vi "Open Motors.vi"(9 "PID Constants":T6={"P Gain"=0.0, "I Gain"=0.0, "D Gain"=0.0, "F Gain"=0.0, "I Zone"=0.0, "Min Output"=-1.0, "Max Output"=1.0}) -> (0 "error out":errorcluster, 1 "Right":T1={"DeviceStatus"={"status"=FALSE, "code"=0, "source"=""}, "Type"=enum."PWM", "PWM"={"PWM Channel"=enum."Invalid", "DeadBand"={"Name"="", "maxPositivePwm"=0, "minPositivePwm"=0, "centerPwm"=0, "maxNegativePwm"=0, "minNegativePwm"=0, "angularRange"=0}}, "CAN"={"Device Number"=0, "SetOutput VI Ref"=variant(refnum<vi> refnum), "GetOutput VI Ref"=variant(refnum<vi> refnum), "Enable VI Ref"=variant(refnum<vi> refnum), "Disable VI Ref"=variant(refnum<vi> refnum), "Data"=variant}, "Invert"=FALSE, "DIO PWM"={"PWM \"Enable\" Channel"=enum."Invalid", "DIOChannel"=enum."Invalid", "PWM Rate"=0.0}}, 2 "Left":T1={"DeviceStatus"={"status"=FALSE, "code"=0, "source"=""}, "Type"=enum."PWM", "PWM"={"PWM Channel"=enum."Invalid", "DeadBand"={"Name"="", "maxPositivePwm"=0, "minPositivePwm"=0, "centerPwm"=0, "maxNegativePwm"=0, "minNegativePwm"=0, "angularRange"=0}}, "CAN"={"Device Number"=0, "SetOutput VI Ref"=variant(refnum<vi> refnum), "GetOutput VI Ref"=variant(refnum<vi> refnum), "Enable VI Ref"=variant(refnum<vi> refnum), "Disable VI Ref"=variant(refnum<vi> refnum), "Data"=variant}, "Invert"=FALSE, "DIO PWM"={"PWM \"Enable\" Channel"=enum."Invalid", "DIOChannel"=enum."Invalid", "PWM Rate"=0.0}}, 3 "WPI Robot":T7={"DevStatus"={"status"=FALSE, "code"=0, "source"=""}, "Motors[]"=[], "Square Inputs"=FALSE, "Max Output"=1.0})   [LabVIEW 2018]
uses:
  <vilib>/Rock Robotics/WPI/RobotDrive/WPI_RobotDriveDevRef.ctl
  <vilib>/Rock Robotics/WPI/MotorControl/WPI_MotorControlDeviceRef.ctl
  <vilib>/Rock Robotics/WPI/MotorControl/WPI_MotorControlType.ctl
  <vilib>/Rock Robotics/SystemInterfaces/DIO/FPGA_DIOPWMChannel.ctl
  <vilib>/Rock Robotics/WPI/PWM/WPI_PWMDeadband.ctl
  <vilib>/Rock Robotics/SystemInterfaces/DIO/FPGA_DIOChannel.ctl
  <vilib>/Rock Robotics/WPI/SafetyOutput/WPI_SafetyOutputConfigMenu.ctl
  <vilib>/Rock Robotics/WPI/ThirdParty/REV Robotics/SPARK MAX/Typedef/Spark MAX Motor Type.ctl
  <vilib>/Rock Robotics/WPI/RobotDrive/WPI_RobotDriveOpen2MotorWithExistingMotors.vi
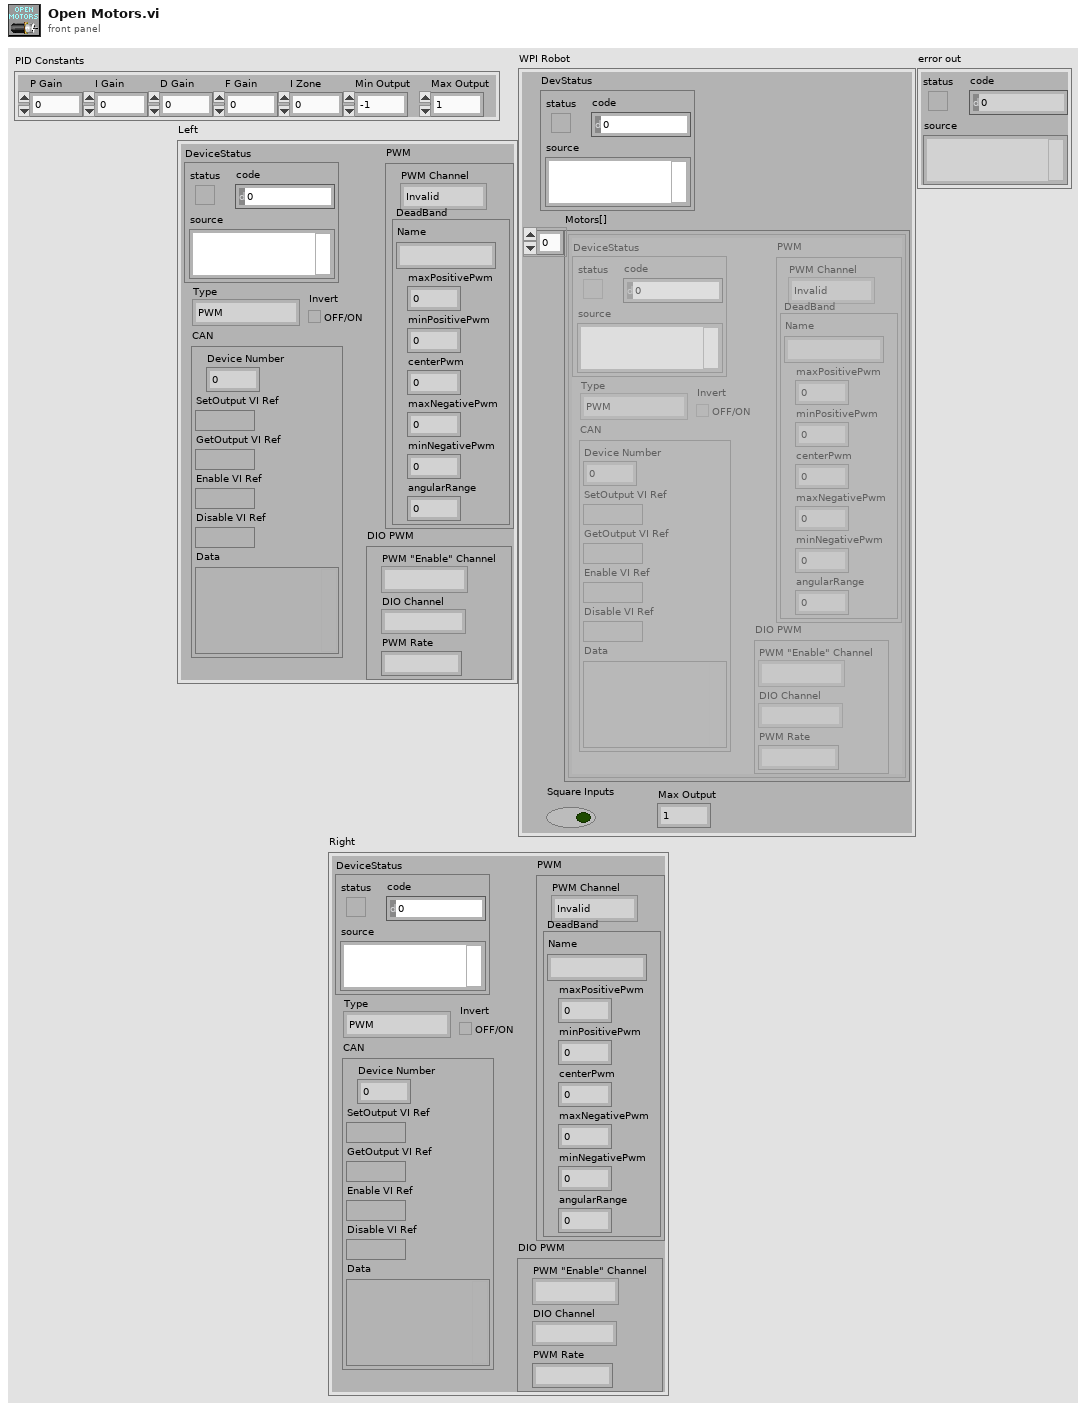
[diagram p1: front panel]
types:
  T1 = typedef "WPI_MotorControlDeviceRef.ctl" = cluster{"DeviceStatus":errorcluster, "Type":T2, "PWM":cluster{"PWM Channel":T3, "DeadBand":T4}, "CAN":cluster{"Device Number":u8, "SetOutput VI Ref":variant, "GetOutput VI Ref":variant, "Enable VI Ref":variant, "Disable VI Ref":variant, "Data":variant}, "Invert":bool, "DIO PWM":cluster{"PWM \"Enable\" Channel":T3, "DIOChannel":T5, "PWM Rate":dbl}}
  T2 = typedef "WPI_MotorControlType.ctl" = enum16{"PWM", "CAN", "DIO PWM"}
  T3 = typedef "FPGA_DIOPWMChannel.ctl" = enum8{"PWM 0", "PWM 1", "PWM 2", "PWM 3", "PWM 4", "PWM 5", "PWM 6", "PWM 7", "PWM 8", "PWM 9", "PWM MXP 0", "PWM MXP 1", "PWM MXP 2", "PWM MXP 3", "PWM MXP 4", "PWM MXP 5", "PWM MXP 6", "PWM MXP 7", "PWM MXP 8", "PWM MXP 9", "Invalid"}
  T4 = typedef "WPI_PWMDeadband.ctl" = cluster{"Name":string, "maxPositivePwm":i32, "minPositivePwm":i32, "centerPwm":i32, "maxNegativePwm":i32, "minNegativePwm":i32, "angularRange":u16}
  T5 = typedef "FPGA_DIOChannel.ctl" = enum8{"DIO 0", "DIO 1", "DIO 2", "DIO 3", "DIO 4", "DIO 5", "DIO 6", "DIO 7", "DIO 8", "DIO 9", "DIO MXP 0", "DIO MXP 1", "DIO MXP 2", "DIO MXP 3", "DIO MXP 4", "DIO MXP 5", "DIO MXP 6", "DIO MXP 7", "DIO MXP 8", "DIO MXP 9", "DIO MXP 10", "DIO MXP 11", "DIO MXP 12", "DIO MXP 13", "DIO MXP 14", "DIO MXP 15", "SPI Port CS1", "SPI Port CS2", "SPI Port CS3", "SPI Port MISO", "SPI Port MOSI", "Invalid"}
  T6 = cluster{"P Gain":dbl, "I Gain":dbl, "D Gain":dbl, "F Gain":dbl, "I Zone":dbl, "Min Output":dbl, "Max Output":dbl}
  T7 = typedef "WPI_RobotDriveDevRef.ctl" = cluster{"DevStatus":errorcluster, "Motors[]":T1[], "Square Inputs":bool, "Max Output":dbl}
  T8 = typedef "Spark MAX Motor Type.ctl" = enum16{"Brushed", "Brushless"}
  T9 = typedef "WPI_SafetyOutputConfigMenu.ctl" = enum16{"Enable", "Disable"}
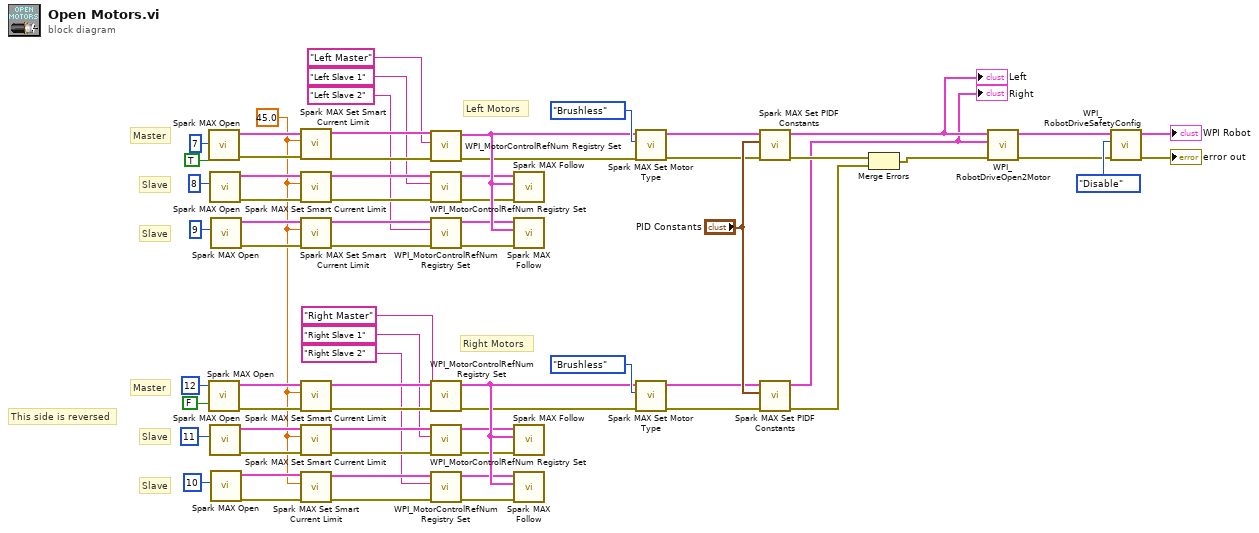
[diagram p0: block diagram]
diagram:
  w22 = 45.0
  # "This side is reversed"
  # "Slave"
  # "Slave"
  # "Master"
  # "Slave"
  # "Slave"
  # "Master"
  # "Right Motors"
  # "Left Motors"
  n1 = call <vilib>:"Spark MAX Open.vi"("Invert"=TRUE, "Device Number"=u8 7) -> ("error out"=w35:errorcluster, "MotorControlDeviceRef"=w38:T1)  [unwired: 8 in]
  n2 = call <vilib>:"Spark MAX Open.vi"("Invert"=FALSE, "Device Number"=u8 12) -> ("error out"=w29:errorcluster, "MotorControlDeviceRef"=w30:T1)  [unwired: 8 in]
  n3 = call <vilib>:"Spark MAX Open.vi"("Device Number"=u8 8) -> ("error out"=w33:errorcluster, "MotorControlDeviceRef"=w34:T1)  [unwired: 9 in]
  n4 = call <vilib>:"Spark MAX Open.vi"("Device Number"=u8 11) -> ("error out"=w25:errorcluster, "MotorControlDeviceRef"=w26:T1)  [unwired: 9 in]
  n5 = call <vilib>:"Spark MAX Open.vi"("Device Number"=u8 9) -> ("error out"=w31:errorcluster, "MotorControlDeviceRef"=w32:T1)  [unwired: 9 in]
  n6 = call <vilib>:"Spark MAX Open.vi"("Device Number"=u8 10) -> ("error out"=w23:errorcluster, "MotorControlDeviceRef"=w24:T1)  [unwired: 9 in]
  n7 = call <vilib>:"Spark MAX Set Smart Current Limit.vi"("error in (no error)"=w35, "Primay Current Limit (80A)"=w22, "MotorControlDeviceRef in"=w38) -> ("error out"=w36:errorcluster, "MotorControlDeviceRef out"=w37:T1)  [unwired: 7 in]
  n8 = call <vilib>:"Spark MAX Set Smart Current Limit.vi"("error in (no error)"=w33, "Primay Current Limit (80A)"=w22, "MotorControlDeviceRef in"=w34) -> ("error out"=w9:errorcluster, "MotorControlDeviceRef out"=w11:T1)  [unwired: 7 in]
  n9 = call <vilib>:"Spark MAX Set Smart Current Limit.vi"("error in (no error)"=w31, "Primay Current Limit (80A)"=w22, "MotorControlDeviceRef in"=w32) -> ("error out"=w5:errorcluster, "MotorControlDeviceRef out"=w7:T1)  [unwired: 7 in]
  n10 = call <vilib>:"Spark MAX Set Smart Current Limit.vi"("error in (no error)"=w29, "Primay Current Limit (80A)"=w22, "MotorControlDeviceRef in"=w30) -> ("error out"=w27:errorcluster, "MotorControlDeviceRef out"=w28:T1)  [unwired: 7 in]
  n11 = call <vilib>:"Spark MAX Set Smart Current Limit.vi"("error in (no error)"=w25, "Primay Current Limit (80A)"=w22, "MotorControlDeviceRef in"=w26) -> ("error out"=w17:errorcluster, "MotorControlDeviceRef out"=w21:T1)  [unwired: 7 in]
  n12 = call <vilib>:"Spark MAX Set Smart Current Limit.vi"("error in (no error)"=w23, "Primay Current Limit (80A)"=w22, "MotorControlDeviceRef in"=w24) -> ("error out"=w15:errorcluster, "MotorControlDeviceRef out"=w19:T1)  [unwired: 7 in]
  n13 = call <vilib>:"WPI_MotorControlRefNum Registry Set.vi"("error in (no error)"=w36, "refnum name"="Left Master", "MotorControlDevRef"=w37) -> ("error out"=w52:errorcluster, "MotorControlDevRef"=w53:T1)  [unwired: 7 in]
  n14 = call <vilib>:"WPI_MotorControlRefNum Registry Set.vi"("error in (no error)"=w9, "refnum name"="Left Slave 1", "MotorControlDevRef"=w11) -> ("error out"=w8:errorcluster, "MotorControlDevRef"=w10:T1)  [unwired: 7 in]
  n15 = call <vilib>:"WPI_MotorControlRefNum Registry Set.vi"("error in (no error)"=w5, "refnum name"="Left Slave 2", "MotorControlDevRef"=w7) -> ("error out"=w4:errorcluster, "MotorControlDevRef"=w6:T1)  [unwired: 7 in]
  n16 = call <vilib>:"WPI_MotorControlRefNum Registry Set.vi"("error in (no error)"=w27, "refnum name"="Right Master", "MotorControlDevRef"=w28) -> ("error out"=w50:errorcluster, "MotorControlDevRef"=w51:T1)  [unwired: 7 in]
  n17 = call <vilib>:"WPI_MotorControlRefNum Registry Set.vi"("error in (no error)"=w17, "refnum name"="Right Slave 1", "MotorControlDevRef"=w21) -> ("error out"=w16:errorcluster, "MotorControlDevRef"=w20:T1)  [unwired: 7 in]
  n18 = call <vilib>:"WPI_MotorControlRefNum Registry Set.vi"("error in (no error)"=w15, "refnum name"="Right Slave 2", "MotorControlDevRef"=w19) -> ("error out"=w12:errorcluster, "MotorControlDevRef"=w18:T1)  [unwired: 7 in]
  n19 = call <vilib>:"Spark MAX Follow.vi"("error in (no error)"=w8, "Master Controller"=w53, "MotorControlDeviceRef"=w10) -> ()  [unwired: 7 in, 2 out]
  n20 = call <vilib>:"Spark MAX Follow.vi"("error in (no error)"=w4, "Master Controller"=w53, "MotorControlDeviceRef"=w6) -> ()  [unwired: 7 in, 2 out]
  n21 = call <vilib>:"Spark MAX Follow.vi"("error in (no error)"=w16, "Master Controller"=w51, "MotorControlDeviceRef"=w20) -> ()  [unwired: 7 in, 2 out]
  n22 = call <vilib>:"Spark MAX Follow.vi"("error in (no error)"=w12, "Master Controller"=w51, "MotorControlDeviceRef"=w18) -> ()  [unwired: 7 in, 2 out]
  n23 = call <vilib>:"Spark MAX Set Motor Type.vi"("error in (no error)"=w52, "Enum"=Spark_MAX_Motor_Type."Brushless", "MotorControlDevRef"=w53) -> ("error out"=w45:errorcluster, "MotorControlDeviceRef"=w46:T1)  [unwired: 7 in]
  n24 = call <vilib>:"Spark MAX Set Motor Type.vi"("error in (no error)"=w50, "Enum"=Spark_MAX_Motor_Type."Brushless", "MotorControlDevRef"=w51) -> ("error out"=w44:errorcluster, "MotorControlDeviceRef"=w47:T1)  [unwired: 7 in]
  n25 = call <vilib>:"Spark MAX Set PIDF Constants.vi"("error in"=w45, "PID Constants"="PID Constants", "MotorControlDeviceRef"=w46) -> ("error out"=w42:errorcluster, "MotorControlDeviceRef"=w41:T1)  [unwired: 7 in]
  "Left" <- w41
  n26 = call <vilib>:"Spark MAX Set PIDF Constants.vi"("error in"=w44, "PID Constants"="PID Constants", "MotorControlDeviceRef"=w47) -> ("error out"=w43:errorcluster, "MotorControlDeviceRef"=w40:T1)  [unwired: 7 in]
  "Right" <- w40
  n27 = Merge Errors(w42, w43) -> (w56:errorcluster)
  n28 = call-poly <vilib>:"WPI_RobotDriveOpen2Motor.vi"("error in (no error)"=w56, "Right Motor Dev Ref"=w40, "Left Motor Dev Ref"=w41) -> ("error out"=w55:errorcluster, "RobotDriveDevRef"=w62:T7)  [unwired: 7 in]
  n29 = call <vilib>:"WPI_RobotDriveSafetyConfig.vi"("error in (no error)"=w55, "mode"=WPI_SafetyOutputConfigMenu."Disable", "RobotDriveDevRef"=w62) -> ("error out"=→"error out":errorcluster, "RobotDriveDevRef"=→"WPI Robot":T7)  [unwired: 7 in]
